vi "Read Macro Steps.vi"(8 "error in (no error)":errorcluster, 10 "Schema Version":string, 11 "refnum":T3) -> (0 "error out":errorcluster, 2 "Macro Steps":T1[](array[typedef]), 3 "refnum out":T3)   [LabVIEW 2023]
doc: "Reads the list of steps from macro config file defined by <B>refnum</B>."
uses:
  <vilib>/Utility/config.llb/Config Data RefNum.ctl
  CTLs/Step V3.ctl
  CTLs/Step Type V3.ctl
  <vilib>/Utility/config.llb/Read Key (I32).vi
  <vilib>/Utility/config.llb/Read Key (String).vi
  <vilib>/Utility/config.llb/Read Key (Boolean).vi
  <vilib>/Utility/config.llb/Read Key (U32).vi
  <vilib>/Utility/error.llb/Error Cluster From Error Code.vi
  <vilib>/ErrorRing/Error Ring.xnode
  <vilib>/Utility/config.llb/NI_LVConfig.lvlib
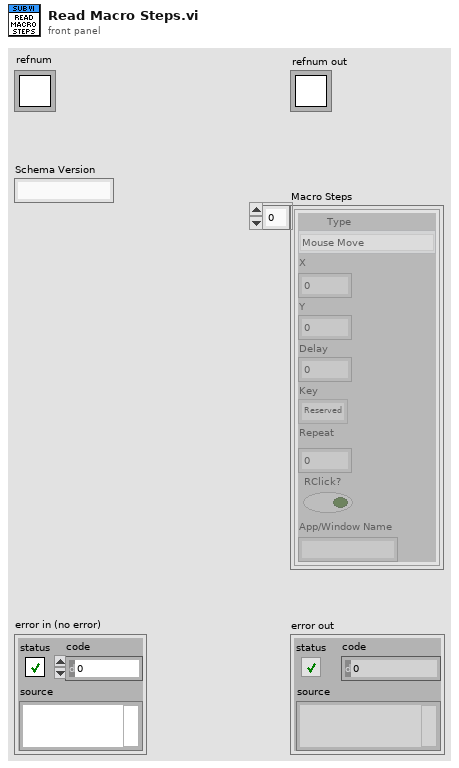
[diagram p1: front panel]
types:
  T1 = typedef "Step V3.ctl" = cluster{"Type":T2, "X":i32, "Y":i32, "Delay":i32, "Key":u8, "Repeat":i32, "RClick?":bool, "App/Window Name":string}
  T2 = typedef "Step Type V3.ctl" = enum16{"Mouse Move", "Mouse Click", "Key Press", "Wait", "Mouse Down", "Mouse Up", "Key Down", "Key Up", "Run Application", "Maximize Window", "Minimize Window", "Close Window", "Bring Window to Front", "Send Window to Back"}
  T3 = typedef "NI_LVConfig.lvlib/Config Data RefNum.ctl" = refnum<k1>
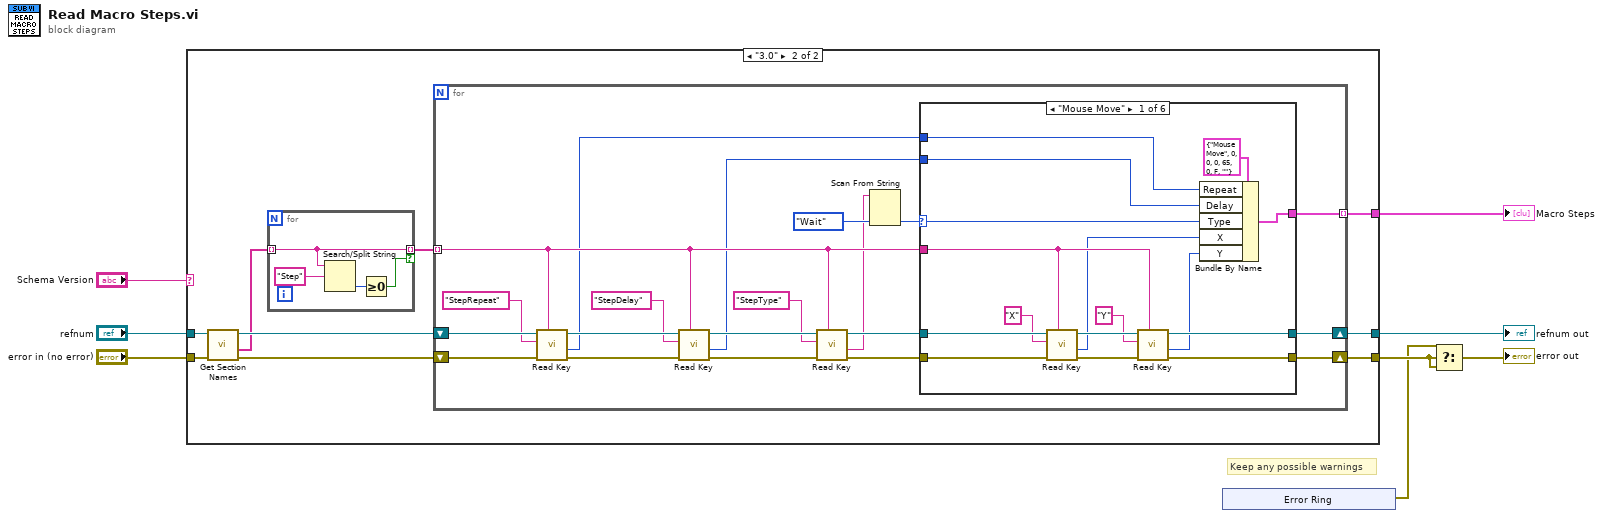
[diagram p0: block diagram]
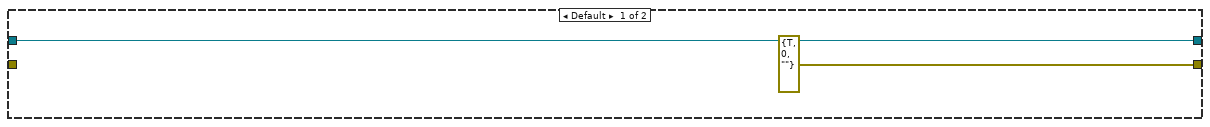
[diagram p2: hidden frame]
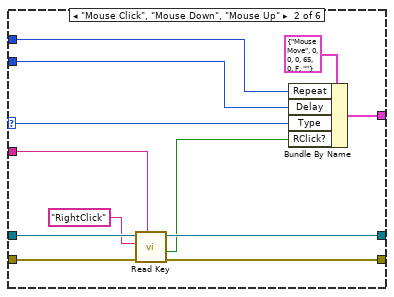
[diagram p3: hidden frame]
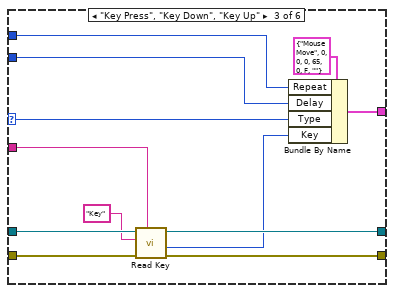
[diagram p4: hidden frame]
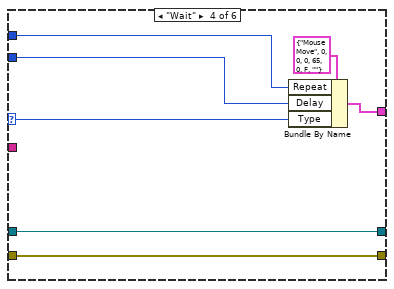
[diagram p5: hidden frame]
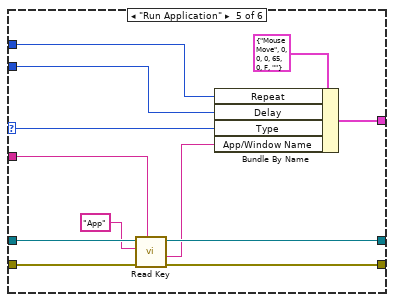
[diagram p6: hidden frame]
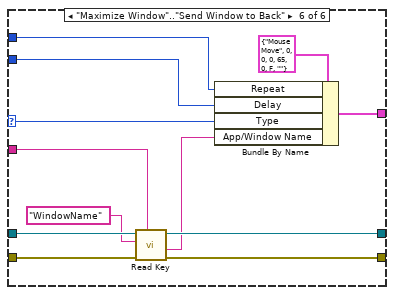
[diagram p7: hidden frame]
diagram:
  # "Keep any possible warnings"
  n1 = case shown="\"3.0\"" "Schema Version" {
    tunnel: "refnum" -> [w10 w16]
    tunnel: [w10 w18] -> w2
    tunnel: [errorcluster {"status"=TRUE, "code"=0, "source"=""} ("error out") w19] -> w8
    tunnel: "error in (no error)" -> [_ w17]
    tunnel: [_ w12] -> w1
    frame Default {
    }
    frame "3.0" {
      n2 = call <vilib>:"Get Section Names.vi"("error in (no error)"=w17, "refnum"=w16) -> ("error out"=w15:errorcluster, "section names"=w13:string[], "refnum out"=w14:T3)  [unwired: 7 in]
      n3 = for {
        tunnel: w13 -> [w111] mode=indexing
        tunnel: [w111] -> w11 mode=indexing if=w112
        n4 = Search/Split String(string=w111, search string/char (-)="Step") -> (offset of match=w113:i32)  [unwired: 1 in, 2 out]
        n5 = Greater Or Equal To 0?(x=w113) -> (x >= 0?=w112:bool)
      }
      n6 = for {
        tunnel: [w30] -> w12 mode=indexing
        shift-right: [w32] -> w19
        shift-left: w15 -> [w36]
        shift-right: [w31] -> w18
        shift-left: w14 -> [w37]
        tunnel: w11 -> [w25] mode=indexing
        n7 = call-poly <vilib>:"Read Key.vi"("section"=w25, "error in (no error)"=w36, "key"="StepRepeat", "refnum"=w37) -> ("error out"=w27:errorcluster, "value"=w21:i32, "refnum out"=w39:T3)  [unwired: 4 in, 1 out]
        n8 = call-poly <vilib>:"Read Key.vi"("section"=w25, "error in (no error)"=w27, "key"="StepDelay", "refnum"=w39) -> ("error out"=w26:errorcluster, "value"=w20:i32, "refnum out"=w38:T3)  [unwired: 4 in, 1 out]
        n9 = call-poly <vilib>:"Read Key.vi"("section"=w25, "error in (no error)"=w26, "key"="StepType", "refnum"=w38) -> ("error out"=w24:errorcluster, "value"=w22:string, "refnum out"=w23:T3)  [unwired: 4 in, 1 out]
        n10 = Scan From String(input string=w22, default 1=Step_Type_V3."Wait" ("Step Type")) -> (output 1=w33:T2)  [unwired: 3 in, 3 out]
        n11 = case shown="\"Mouse Move\"" w33 {
          selector: w33 -> [w45 w62 w74 w85 w93 w105]
          tunnel: w24 -> [w54 w67 w79 w82 w98 w110]
          tunnel: w23 -> [w53 w66 w78 w83 w97 w109]
          tunnel: w25 -> [w49 w64 w76 _ w95 w107]
          tunnel: [w48 w58 w71 w82 w90 w102] -> w32
          tunnel: [w47 w60 w72 w83 w91 w103] -> w31
          tunnel: [w42 w61 w73 w84 w92 w104] -> w30
          tunnel: w21 -> [w40 w56 w68 w80 w87 w99]
          tunnel: w20 -> [w41 w57 w69 w81 w88 w100]
          frame "Mouse Move" {
            n12 = call-poly <vilib>:"Read Key.vi"("section"=w49, "error in (no error)"=w54, "key"="X", "refnum"=w53) -> ("error out"=w50:errorcluster, "value"=w44:i32, "refnum out"=w55:T3)  [unwired: 4 in, 1 out]
            n13 = call-poly <vilib>:"Read Key.vi"("section"=w49, "error in (no error)"=w50, "key"="Y", "refnum"=w55) -> ("error out"=w48:errorcluster, "value"=w43:i32, "refnum out"=w47:T3)  [unwired: 4 in, 1 out]
            n14 = Bundle By Name(cluster=T1 {"Type"=enum."Mouse Move", "X"=0, "Y"=0, "Delay"=0, "Key"=65, "Repeat"=0, "RClick?"=FALSE, "App/Window Name"=""} ("Step"), "Repeat"=w40, "Delay"=w41, "Type"=w45, "X"=w44, "Y"=w43) -> (w42:T1)
          }
          frame "Mouse Click", "Mouse Down", "Mouse Up" {
            n15 = call-poly <vilib>:"Read Key.vi"("section"=w64, "error in (no error)"=w67, "key"="RightClick", "refnum"=w66) -> ("error out"=w58:errorcluster, "value"=w59:bool, "refnum out"=w60:T3)  [unwired: 4 in, 1 out]
            n16 = Bundle By Name(cluster=T1 {"Type"=enum."Mouse Move", "X"=0, "Y"=0, "Delay"=0, "Key"=65, "Repeat"=0, "RClick?"=FALSE, "App/Window Name"=""} ("Step"), "Repeat"=w56, "Delay"=w57, "Type"=w62, "RClick?"=w59) -> (w61:T1)
          }
          frame "Key Press", "Key Down", "Key Up" {
            n17 = call-poly <vilib>:"Read Key.vi"("section"=w76, "error in (no error)"=w79, "key"="Key", "refnum"=w78) -> ("error out"=w71:errorcluster, "value"=w70:u32, "refnum out"=w72:T3)  [unwired: 4 in, 1 out]
            n18 = Bundle By Name(cluster=T1 {"Type"=enum."Mouse Move", "X"=0, "Y"=0, "Delay"=0, "Key"=65, "Repeat"=0, "RClick?"=FALSE, "App/Window Name"=""} ("Step"), "Repeat"=w68, "Delay"=w69, "Type"=w74, "Key"=w70) -> (w73:T1)
          }
          frame "Wait" {
            n19 = Bundle By Name(cluster=T1 {"Type"=enum."Mouse Move", "X"=0, "Y"=0, "Delay"=0, "Key"=65, "Repeat"=0, "RClick?"=FALSE, "App/Window Name"=""} ("Step"), "Repeat"=w80, "Delay"=w81, "Type"=w85) -> (w84:T1)
          }
          frame "Run Application" {
            n20 = call-poly <vilib>:"Read Key.vi"("section"=w95, "error in (no error)"=w98, "key"="App", "refnum"=w97) -> ("error out"=w90:errorcluster, "value"=w89:string, "refnum out"=w91:T3)  [unwired: 4 in, 1 out]
            n21 = Bundle By Name(cluster=T1 {"Type"=enum."Mouse Move", "X"=0, "Y"=0, "Delay"=0, "Key"=65, "Repeat"=0, "RClick?"=FALSE, "App/Window Name"=""} ("Step"), "Repeat"=w87, "Delay"=w88, "Type"=w93, "App/Window Name"=w89) -> (w92:T1)
          }
          frame "Maximize Window".."Send Window to Back" {
            n22 = call-poly <vilib>:"Read Key.vi"("section"=w107, "error in (no error)"=w110, "key"="WindowName", "refnum"=w109) -> ("error out"=w102:errorcluster, "value"=w101:string, "refnum out"=w103:T3)  [unwired: 4 in, 1 out]
            n23 = Bundle By Name(cluster=T1 {"Type"=enum."Mouse Move", "X"=0, "Y"=0, "Delay"=0, "Key"=65, "Repeat"=0, "RClick?"=FALSE, "App/Window Name"=""} ("Step"), "Repeat"=w99, "Delay"=w100, "Type"=w105, "App/Window Name"=w101) -> (w104:T1)
          }
        }
      }
    }
  }
  "refnum out" <- w2
  "Macro Steps" <- w1
  n24 = xnode "Error Ring"() -> ("error out"=w7:errorcluster)
  n25 = Select(t=w7, s=w8, f=w8) -> (s? t:f=→"error out":errorcluster)
